vi "InitiateGeneration.vi"(8 "error in (no error)":errorcluster, 11 "ClassIn":refnum<class "NiPxi6733.lvclass">) -> (0 "error out":errorcluster, 3 "ClassOut":refnum<class "NiPxi6733.lvclass">)   [LabVIEW 2014, in "FGenPlugins.lvlib" / "NiPxi6733.lvclass"]
uses:
  NiPxi6733.lvclass
  MyPluginBaseClass/NISTFGenPluginsBase.lvclass/NISTFGenPluginsBase.ctl
  MyPluginBaseClass/Accessors/Write Timestamp.vi
  <vilib>/DAQmx/write.llb/DAQmx Write (Analog 1D Wfm NChan NSamp).vi
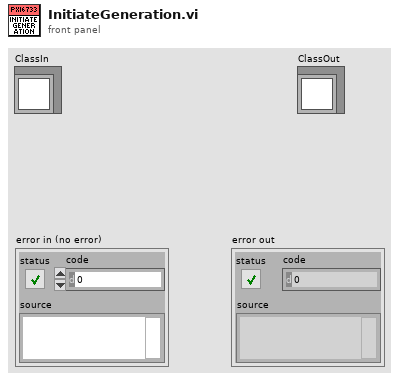
[diagram p1: front panel]
types:
  T1 = typedef "FGenPlugins.lvlib/NISTFGenPluginsBase.lvclass/ChannelParamElement.ctl" = cluster{"sName":string, "eOperateMode":u16, "bEnabled":bool, "eOutputMode":u16, "iIndex":i32, "iNameBufferSize":i32, "fGain":dbl}
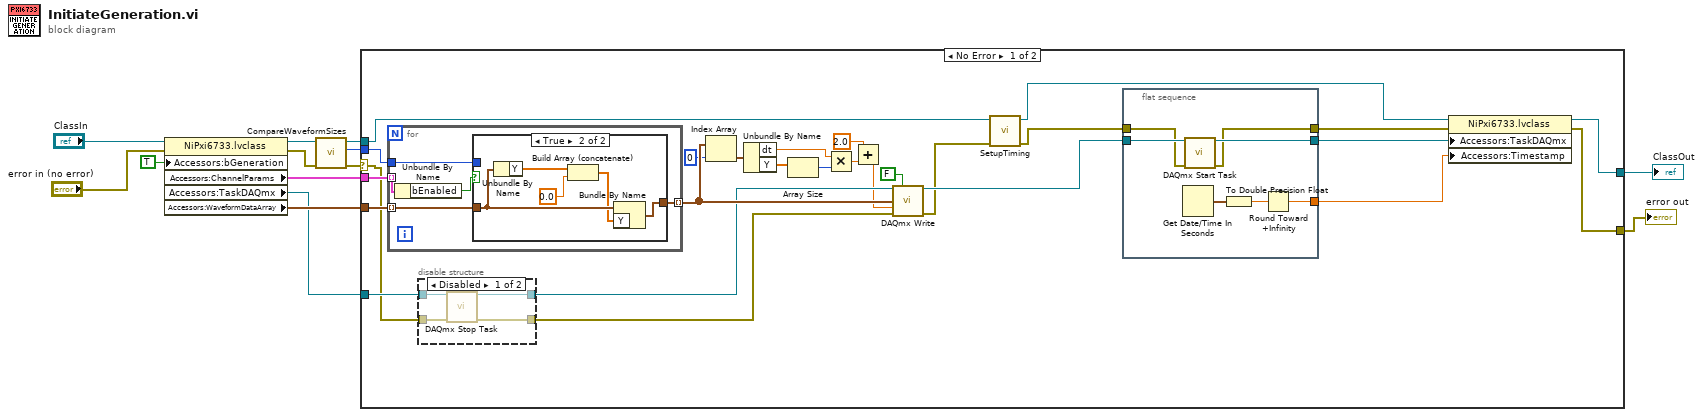
[diagram p0: block diagram]
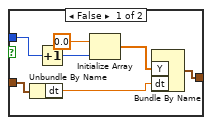
[diagram p3: hidden frame]
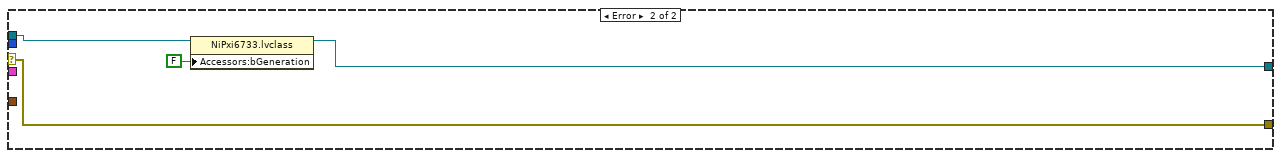
[diagram p4: hidden frame]
diagram:
  n1 = property class="NiPxi6733.lvclass"(reference="ClassIn", error in="error in (no error)", "Accessors:bGeneration"=TRUE ("bGeneration")) -> (reference out=w5:refnum<class "NiPxi6733.lvclass">, error out=w6:errorcluster, "Accessors:ChannelParams"=w7:T1[], "Accessors:TaskDAQmx"=w2:refnum<k21>, "Accessors:WaveformDataArray"=w3:waveform(dbl)[])
  n2 = call "CompareWaveformSizes.vi"("error in (no error)"=w6, "ClassIn"=w5) -> ("error out"=w1:errorcluster, "WaveformSize"=w8:i32, "ClassOut"=w4:refnum<class "NiPxi6733.lvclass">)  [unwired: 7 in]
  n3 = case shown="No Error" w1 {
    selector: w1 -> [w28 w71]
    tunnel: w8 -> [w40 _]
    tunnel: w7 -> [w39 _]
    tunnel: [w21 w72] -> w10
    tunnel: [w22 w71] -> w11
    tunnel: w4 -> [w17 w74]
    tunnel: w3 -> [w38 _]
    tunnel: w2 -> [w29 _]
    frame No Error {
      n4 = for {
        tunnel: w39 -> [w58] mode=indexing
        tunnel: w38 -> [w55] mode=indexing
        tunnel: [w57] -> w37 mode=indexing
        tunnel: w40 -> [w56]
        n5 = Unbundle By Name(w58) -> ("bEnabled"=w54:bool)
        n6 = case shown="True" w54 {
          tunnel: w55 -> [w65 w69]
          tunnel: [w63 w70] -> w57
          tunnel: w56 -> [w62 _]
          frame False {
            n7 = Unbundle By Name(w65) -> ("dt"=w64:dbl)
            n8 = Increment(x=w62) -> (x+1=w59:i32)
            n9 = Initialize Array(0.0, w59) -> (w60:dbl[])
            n10 = Bundle By Name("Y"=w60, "dt"=w64) -> (w63:waveform(dbl))  [unwired: 1 in]
          }
          frame True {
            n11 = Unbundle By Name(w69) -> ("Y"=w67:dbl[])
            n12 = Build Array (concatenate)(w67, 0.0 ("new element/subarray")) -> (w66:dbl[])
            n13 = Bundle By Name(cluster=w69, "Y"=w66) -> (w70:waveform(dbl))
          }
        }
      }
      n14 = disable-structure shown="Disabled" {
        disable-tunnel: w29 -> [w51 w53]
        disable-tunnel: [w50 w53] -> w27
        disable-tunnel: w28 -> [w49 w52]
        disable-tunnel: [w48 w52] -> w26
        frame Disabled {
          n15 = call <vilib>:"DAQmx Stop Task.vi"("task/channels in"=w51, "error in"=w49) -> ("task out"=w50:refnum<k21>, "error out"=w48:errorcluster)  [unwired: 12 in]
        }
        frame Enabled {
        }
      }
      n16 = Index Array(array=w37, index=0) -> (element=w35:waveform(dbl))
      n17 = Unbundle By Name(w35) -> ("dt"=w32:dbl, "Y"=w34:dbl[])
      n18 = Array Size(array=w34) -> (size(s)=w33:i32)
      n19 = Multiply(x=w32, y=w33) -> (x*y=w31:dbl)
      n20 = Add(x=2.0, y=w31) -> (x+y=w18:dbl)
      n21 = call-poly <vilib>:"DAQmx Write.vi"("task/channels in"=w27, "auto start"=FALSE, "data"=w37, "timeout"=w18, "error in"=w26) -> ("task out"=w25:refnum<k21>, "error out"=w15:errorcluster)  [unwired: 8 in, 1 out]
      n22 = call "SetupTiming.vi"("error in (no error)"=w15, "ClassIn"=w17) -> ("error out"=w14:errorcluster, "ClassOut"=w16:refnum<class "NiPxi6733.lvclass">)  [unwired: 8 in]
      n23 = flat-sequence {
        tunnel: w25 -> [w47]
        tunnel: w14 -> [w46]
        tunnel: [w45] -> w24
        tunnel: [w44] -> w23
        tunnel: [w41] -> w20
        frame #0 {
          n24 = Get Date/Time In Seconds() -> (seconds since 1Jan1904=w43:timestamp)
          n25 = call <vilib>:"DAQmx Start Task.vi"("task/channels in"=w47, "error in"=w46) -> ("task out"=w45:refnum<k21>, "error out"=w44:errorcluster)  [unwired: 12 in]
          n26 = To Double Precision Float(number=w43) -> (double precision float=w42:dbl)
          n27 = Round Toward +Infinity(x=w42) -> (ceil(x): smallest int >= x=w41:dbl)
        }
      }
      n28 = property class="NiPxi6733.lvclass"(reference=w16, error in=w23, "Accessors:TaskDAQmx"=w24, "Accessors:Timestamp"=w20) -> (reference out=w21:refnum<class "NiPxi6733.lvclass">, error out=w22:errorcluster)
    }
    frame Error {
      n29 = property class="NiPxi6733.lvclass"(reference=w74, "Accessors:bGeneration"=FALSE ("bGeneration")) -> (reference out=w72:refnum<class "NiPxi6733.lvclass">)  [unwired: 1 in, 1 out]
    }
  }
  "error out" <- w11
  "ClassOut" <- w10
